vi "snap_qrcode.vi"() -> ()   [LabVIEW 2018]
panel:
  out "Input QR Code":picture
  out "Output QR Code":picture
  out "return value":cluster{"found":i32, "decode data":string}
  in  "Output image filename":string="decode.png"
  in  "QR Code Image Path":path=path "hello.png"
  # "Free QR code generator website"
  # "https://www.the-qrcode-generator.com/"
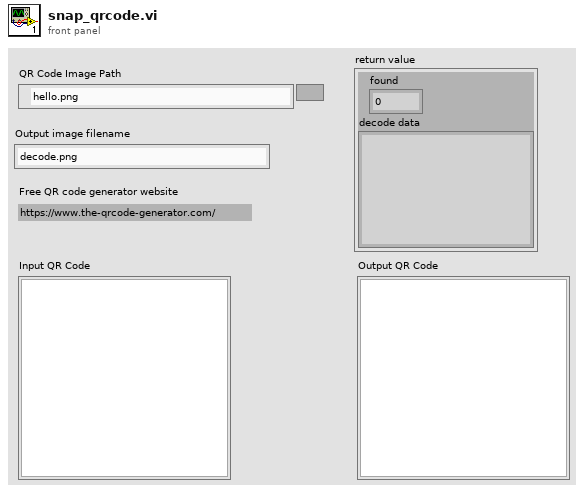
[diagram p1: front panel]
types:
  T1 = typedef "imagedata.ctl" = cluster{"image type":i32, "image depth":i32, "image":u8[], "mask":u8[], "colors":u32[], "Rectangle":cluster{"left":i16, "top":i16, "right":i16, "bottom":i16}}
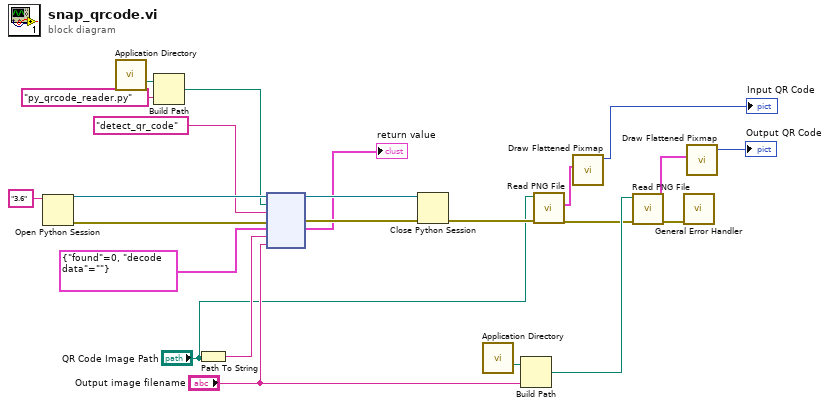
[diagram p0: block diagram]
diagram:
  n1 = Open Python Session(python version="3.6" ("Python version")) -> (session out=w22:refnum<k35>, error out=w20:errorcluster)  [unwired: 2 in]
  n2 = call <vilib>:"Application Directory.vi"() -> ("Application Directory"=w8:path)
  n3 = Build Path(base path=w8, name or relative path="py_qrcode_reader.py" ("module filename")) -> (appended path=w6:path)
  n4 = Path To String(path="QR Code Image Path") -> (string=w16:string)
  n5 = node(w22, w6, "detect_qr_code" ("function name"), w20, cluster{"found":i32, "decode data":string} {"found"=0, "decode data"=""}, w16, "Output image filename") -> (w21:refnum<k35>, w19:errorcluster, →"return value":cluster{"found":i32, "decode data":string})  [unwired: 2 in, 2 out]
  n6 = Close Python Session(session in=w21, error in=w19) -> (11:w5:errorcluster)
  n7 = call <vilib>:"Application Directory.vi"() -> ("Application Directory"=w14:path)
  n8 = Build Path(base path=w14, name or relative path="Output image filename") -> (appended path=w12:path)
  n9 = call <vilib>:"Read PNG File.vi"("error in (no error)"=w5, "path to PNG file"="QR Code Image Path") -> ("error out"=w4:errorcluster, "image data"=w2:T1)  [unwired: 7 in, 1 out]
  n10 = call <vilib>:"Draw Flattened Pixmap.vi"("image data"=w2) -> ("new picture"=→"Input QR Code":picture)  [unwired: 8 in]
  n11 = call <vilib>:"Read PNG File.vi"("error in (no error)"=w4, "path to PNG file"=w12) -> ("error out"=w9:errorcluster, "image data"=w11:T1)  [unwired: 7 in, 1 out]
  n12 = call <vilib>:"General Error Handler.vi"("error in (no error)"=w9) -> ()  [unwired: 10 in, 5 out]
  n13 = call <vilib>:"Draw Flattened Pixmap.vi"("image data"=w11) -> ("new picture"=→"Output QR Code":picture)  [unwired: 8 in]
